vi "题目7.vi"() -> ()   [LabVIEW 2017]
panel:
  out "所需时间":dbl
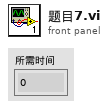
[diagram p1: front panel]
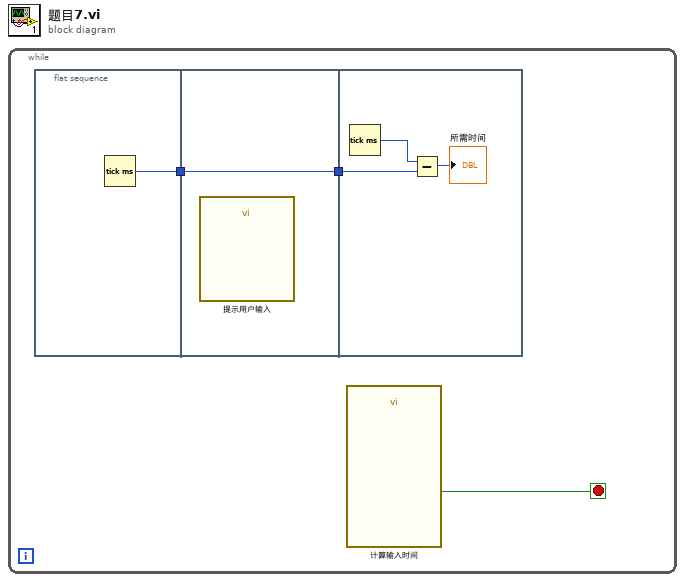
[diagram p0: block diagram]
diagram:
  n1 = while {
    stop <- w3 stop-if-true
    n2 = flat-sequence {
      tunnel: [w4] -> w2
      tunnel: [w5] -> w1
      tunnel: w2 -> [w5]
      tunnel: w1 -> [w8]
      frame #0 {
        n3 = Tick Count (ms)() -> (millisecond timer value=w4:u32)
      }
      frame #1 {
        n4 = call "提示用户输入"() -> ()  [unwired: 17 in, 3 out]
      }
      frame #2 {
        n5 = Tick Count (ms)() -> (millisecond timer value=w7:u32)
        n6 = Subtract(x=w7, y=w8) -> (x-y=→"所需时间":u32)
      }
    }
    n7 = call "计算输入时间"() -> ("确定"=w3:bool)  [unwired: 10 in, 1 out]
  }
